vi "ALTS-2015 Set Light Indicators_Idle.vi"(8 "error in (no error)":errorcluster) -> (0 "error out":errorcluster)   [LabVIEW 2013]
doc: "Copyright © 2005, Soliton Technologies.\nAll rights reserved."
uses:
  Controls/ALTS-2015 LV2GBL Options.ctl
  Controls/ALTS-2015 Station Cluster.ctl
  Controls/ALTS-2015 Digital Output Options.ctl
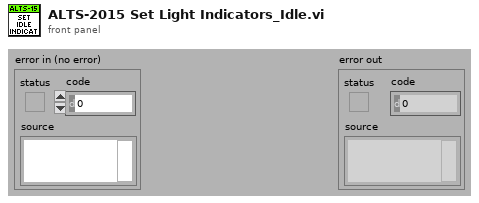
[diagram p1: front panel]
types:
  T1 = typedef "ALTS-2015 LV2GBL Options.ctl" = enum16{"Read all", "Write all"}
  T2 = typedef "ALTS-2015 Digital Output Options.ctl" = enum16{"Idle", "Test Running", "Pass", "Fail"}
  T3 = typedef "ALTS-2015 Station Cluster.ctl" = enum16{"Station 1", "Station 2", "Station 3", "Station 4"}
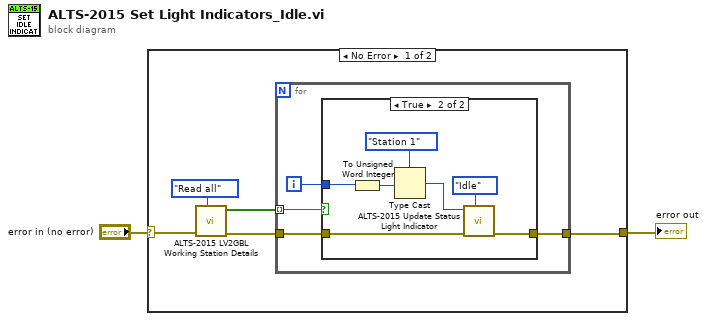
[diagram p0: block diagram]
diagram:
  n1 = case shown="No Error" "error in (no error)" {
    selector: "error in (no error)" -> [w6 w20]
    tunnel: [w7 w20] -> w1
    frame No Error {
      n2 = call "ALTS-2015 LV2GBL Working Station Details.vi"("Options"=ALTS-2015_LV2GBL_Options."Read all", "error in"=w6) -> ("error out"=w5:errorcluster, "Station  Enable Array"=w4:bool[])  [unwired: 8 in]
      n3 = for {
        tunnel: w5 -> [w11]
        tunnel: [w10] -> w7
        tunnel: w4 -> [w8] mode=indexing
        i -> [w9]
        n4 = case shown="True" w8 {
          tunnel: w11 -> [w12 w19]
          tunnel: [w12 w18] -> w10
          tunnel: w9 -> [_ w17]
          frame False {
          }
          frame True {
            n5 = To Unsigned Word Integer(number=w17) -> (unsigned 16bit integer=w15:u16)
            n6 = Type Cast(type=ALTS-2015_Station_Cluster."Station 1" ("Station Cluster"), x=w15) -> (*(type *) &x=w14:T3)
            n7 = call "ALTS-2015 Update Status Light Indicator.vi"("DO Options"=ALTS-2015_Digital_Output_Options."Idle", "error in"=w19, "Station Cluster"=w14) -> ("error out"=w18:errorcluster)  [unwired: 8 in]
          }
        }
      }
    }
    frame Error {
    }
  }
  "error out" <- w1
